vi "TurretChooseAngle2.vi"() -> ()   [LabVIEW 2019]
panel:
  in  "Hysterisis":dbl
  in  "Current Turret Azimuth [0, 360]":dbl(knob)
  out "Working Angular Delta":dbl
  in  "Dead Zone Position B":dbl=100.0
  in  "Dead Zone Position A":dbl=80.0
  in  "Heading to Target Delta (best) [-180,+180]":dbl
  # "Counter Clock Wise = +\nClock Wise = -"
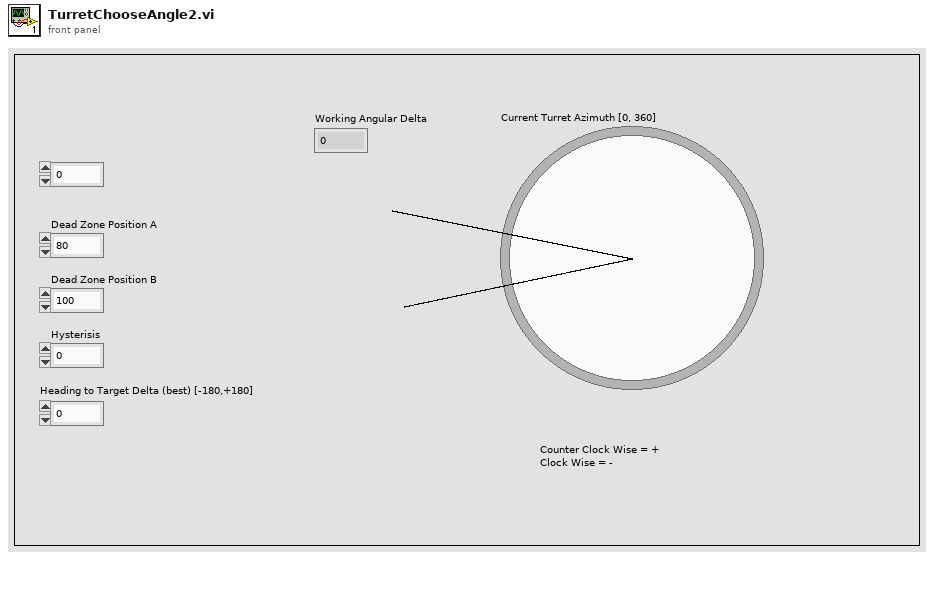
[diagram p1: front panel]
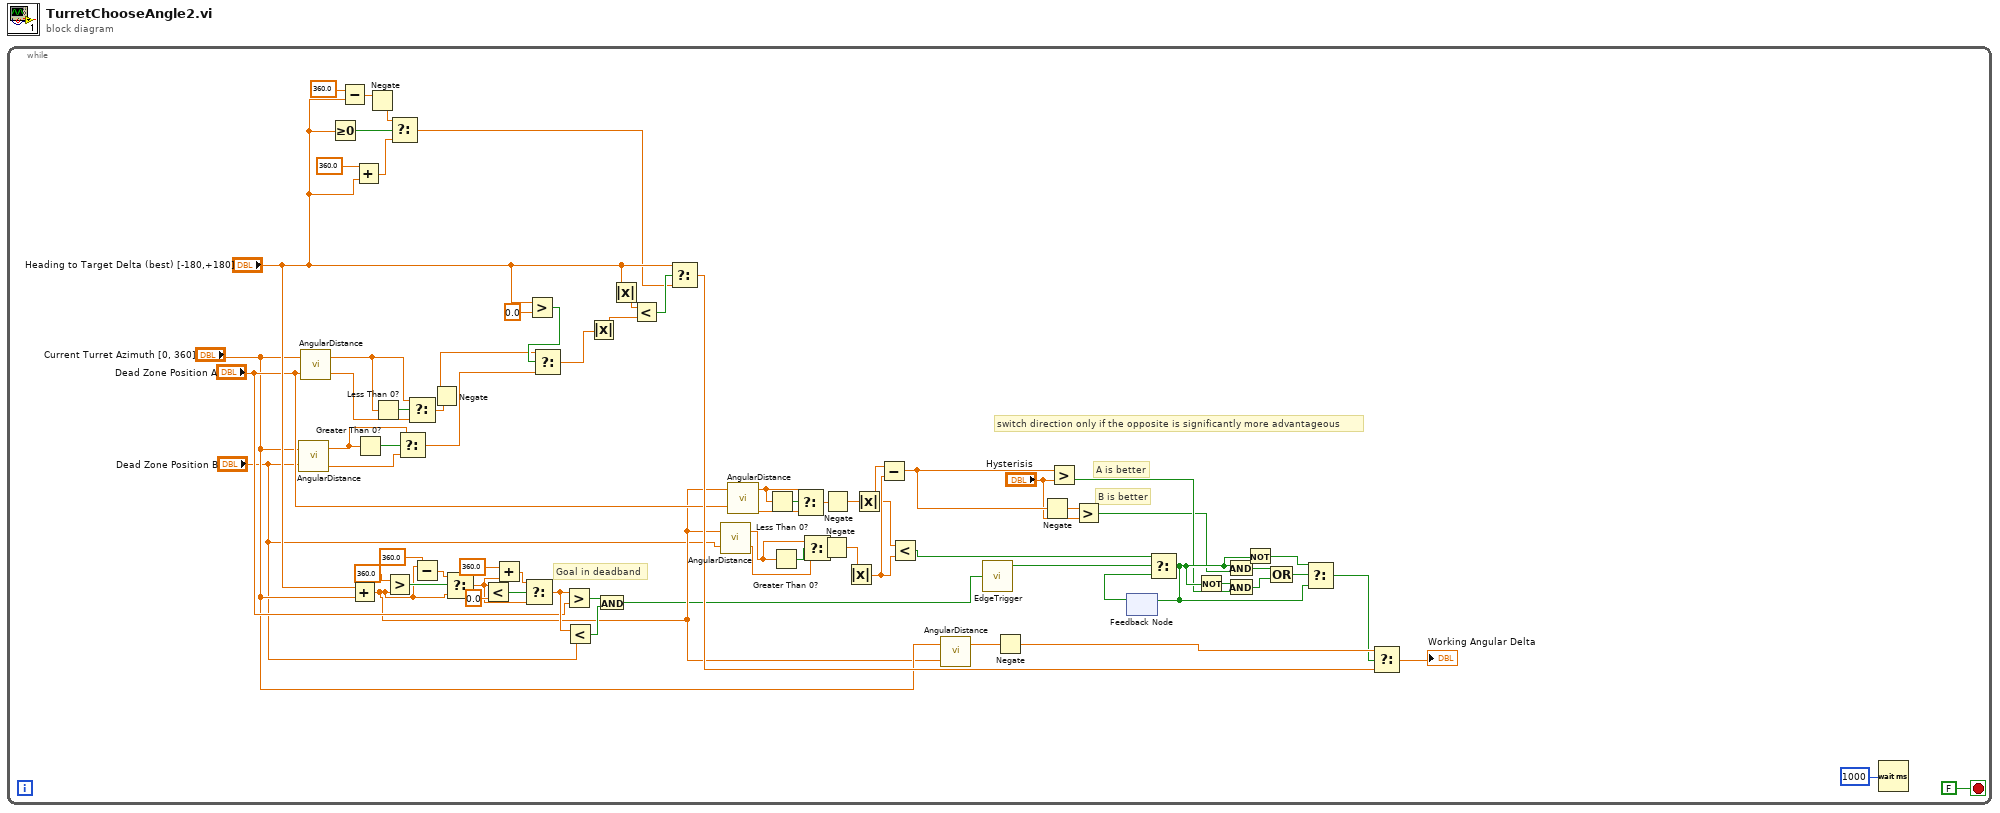
[diagram p0: block diagram]
diagram:
  n1 = while {
    stop <- FALSE stop-if-true
    # "switch direction only if the opposite is significantly more advantageous"
    # "B is better"
    # "A is better"
    # "Goal in deadband"
    n2 = call "AngularDistance.vi"("Goal Angle (deg) [0,360]"="Dead Zone Position B", "Current Angle (deg) [-Inf,+Inf]"="Current Turret Azimuth [0, 360]") -> ("Alternate Signed Angular Distance (deg) [-180,+180]"=w71:dbl, "Signed Angular Distance (deg) [-180,+180]"=w72:dbl)
    n3 = call "AngularDistance.vi"("Goal Angle (deg) [0,360]"="Dead Zone Position A", "Current Angle (deg) [-Inf,+Inf]"="Current Turret Azimuth [0, 360]") -> ("Alternate Signed Angular Distance (deg) [-180,+180]"=w73:dbl, "Signed Angular Distance (deg) [-180,+180]"=w60:dbl)
    n4 = Greater Or Equal To 0?(x="Heading to Target Delta (best) [-180,+180]") -> (x >= 0?=w69:bool)
    n5 = Subtract(x=360.0, y="Heading to Target Delta (best) [-180,+180]") -> (x-y=w64:dbl)
    n6 = Add(x="Heading to Target Delta (best) [-180,+180]", y="Current Turret Azimuth [0, 360]") -> (x+y=w31:dbl)
    n7 = Add(x=360.0, y="Heading to Target Delta (best) [-180,+180]") -> (x+y=w62:dbl)
    n8 = Greater Than 0?(x=w72) -> (x > 0?=w56:bool)
    n9 = Negate(x=w64) -> (-x=w63:dbl)
    n10 = Less Than 0?(x=w60) -> (x < 0?=w57:bool)
    n11 = Greater?(x=360.0, y=w31) -> (0:w54:bool)
    n12 = Select(t=w63, s=w69, f=w62) -> (s? t:f=w16:dbl)
    n13 = Select(t=w72, s=w56, f=w71) -> (s? t:f=w17:dbl)
    n14 = Select(t=w60, s=w57, f=w73) -> (s? t:f=w67:dbl)
    n15 = Subtract(x=w31, y=360.0) -> (x-y=w52:dbl)
    n16 = Negate(x=w67) -> (-x=w18:dbl)
    n17 = Select(t=w52, s=w54, f=w31) -> (s? t:f=w47:dbl)
    n18 = Less?(x=w47, y=0.0) -> (x < y?=w50:bool)
    n19 = Add(x=360.0, y=w47) -> (x+y=w49:dbl)
    n20 = Select(t=w49, s=w50, f=w47) -> (s? t:f=w44:dbl)
    n21 = Greater?(x="Heading to Target Delta (best) [-180,+180]", y=0.0) -> (0:w58:bool)
    n22 = Select(t=w18, s=w58, f=w17) -> (s? t:f=w42:dbl)
    n23 = Greater?(x=w44, y="Dead Zone Position A") -> (0:w46:bool)
    n24 = Less?(x=w44, y="Dead Zone Position B") -> (x < y?=w45:bool)
    n25 = Absolute Value(x=w42) -> (abs(x)=w65:dbl)
    n26 = And(x=w46, y=w45) -> (x .and. y?=w11:bool)
    n27 = Absolute Value(x="Heading to Target Delta (best) [-180,+180]") -> (abs(x)=w66:dbl)
    n28 = Less?(x=w66, y=w65) -> (x < y?=w70:bool)
    n29 = Select(t="Heading to Target Delta (best) [-180,+180]", s=w70, f=w16) -> (s? t:f=w43:dbl)
    n30 = call "AngularDistance.vi"("Goal Angle (deg) [0,360]"="Dead Zone Position B", "Current Angle (deg) [-Inf,+Inf]"=w31) -> ("Alternate Signed Angular Distance (deg) [-180,+180]"=w22:dbl, "Signed Angular Distance (deg) [-180,+180]"=w23:dbl)
    n31 = call "AngularDistance.vi"("Goal Angle (deg) [0,360]"="Dead Zone Position A", "Current Angle (deg) [-Inf,+Inf]"=w31) -> ("Alternate Signed Angular Distance (deg) [-180,+180]"=w39:dbl, "Signed Angular Distance (deg) [-180,+180]"=w38:dbl)
    n32 = Less Than 0?(x=w38) -> (x < 0?=w37:bool)
    n33 = Greater Than 0?(x=w23) -> (x > 0?=w36:bool)
    n34 = Select(t=w38, s=w37, f=w39) -> (s? t:f=w25:dbl)
    n35 = Select(t=w23, s=w36, f=w22) -> (s? t:f=w24:dbl)
    n36 = Negate(x=w24) -> (-x=w20:dbl)
    n37 = Negate(x=w25) -> (-x=w19:dbl)
    n38 = Absolute Value(x=w20) -> (abs(x)=w28:dbl)
    n39 = Absolute Value(x=w19) -> (abs(x)=w27:dbl)
    n40 = Subtract(x=w27, y=w28) -> (x-y=w30:dbl)
    n41 = Less?(x=w27, y=w28) -> (x < y?=w12:bool)
    n42 = call "AngularDistance.vi"("Goal Angle (deg) [0,360]"=w31, "Current Angle (deg) [-Inf,+Inf]"="Current Turret Azimuth [0, 360]") -> ("Signed Angular Distance (deg) [-180,+180]"=w33:dbl)  [unwired: 1 out]
    n43 = call "EdgeTrigger.vi"("Input Signal"=w11) -> ("Rising Edge Trigger"=w13:bool)  [unwired: 2 out]
    n44 = Negate(x=w33) -> (-x=w40:dbl)
    n45 = Negate(x=w30) -> (-x=w29:dbl)
    n46 = Greater?(x=w30, y="Hysterisis") -> (0:w3:bool)
    n47 = Greater?(x=w29, y="Hysterisis") -> (0:w2:bool)
    n48 = feedback #1() -> (w14:bool)  [unwired: 1 in]
    n49 = Select(t=w12, s=w13, f=w14) -> (s? t:f=w6:bool)
    n50 = feedback-in #1(w6) -> ()
    n51 = Not(x=w6) -> (.not. x?=w8:bool)
    n52 = And(x=w6, y=w2) -> (x .and. y?=w10:bool)
    n53 = And(x=w8, y=w3) -> (x .and. y?=w9:bool)
    n54 = Not(x=w6) -> (.not. x?=w5:bool)
    n55 = Compound Arithmetic op=OR(w10, w9) -> (w7:bool)
    n56 = Select(t=w5, s=w7, f=w6) -> (s? t:f=w4:bool)
    n57 = Select(t=w40, s=w4, f=w43) -> (s? t:f=→"Working Angular Delta":dbl)
    n58 = Wait (ms)(milliseconds to wait=u32 1000) -> ()  [unwired: 1 out]
  }
